vi "Read Width.vi"(8 "error in (no error)":errorcluster, 11 "CollisionGrid in":refnum<class "CollisionGrid.lvclass">) -> (0 "error out":errorcluster, 2 "Width":i8, 3 "CollisionGrid out":refnum<class "CollisionGrid.lvclass">)   [LabVIEW 2022 SP3, in "CollisionGrid.lvclass"]
uses:
  CollisionGrid.lvclass
  CollisionGrid.lvclass/CollisionGrid.ctl
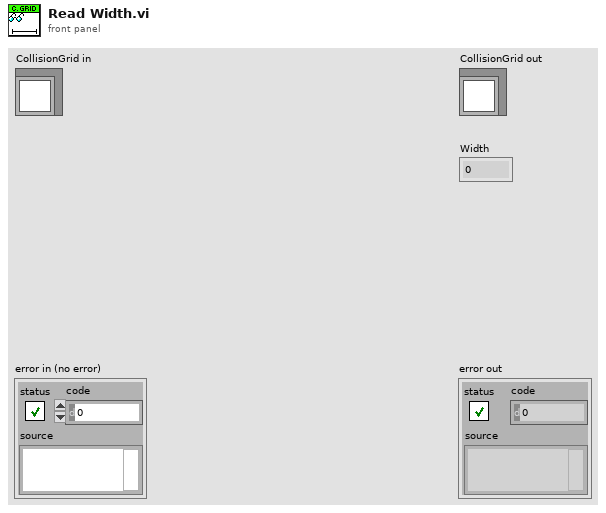
[diagram p1: front panel]
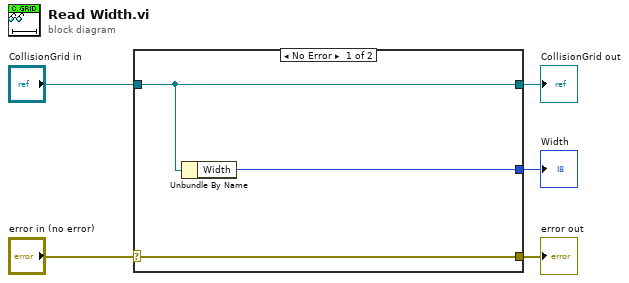
[diagram p0: block diagram]
diagram:
  n1 = case shown="No Error" "error in (no error)" {
    selector: "error in (no error)" -> [w8 w9]
    tunnel: [w8 w9] -> w4
    tunnel: [w7 w10] -> w2
    tunnel: "CollisionGrid in" -> [w7 w10]
    tunnel: [w6 _] -> w1
    frame No Error {
      n2 = Unbundle By Name(w7) -> ("Width"=w6:i8)
    }
    frame Error {
    }
  }
  "error out" <- w4
  "CollisionGrid out" <- w2
  "Width" <- w1
